vi "translate_to_from_byte_array.vi"(0 "actions":T1, 5 "byte_array (in)":u8[](array[numeric]), 7 "string (in)":string) -> (6 "byte_array (out)":u8[](array[numeric]), 8 "string (out)":string)   [LabVIEW 2013, in "common.lvlib"]
doc: "Converts a String to Byte Array and Byte Array to String for ease of communication with Performax hardware.\n\nProduced By:\n\n<B>Kod Integrations, LLC</B>\n4835 Marianne Drive\nMount Airy, MD 21771\nhttp://www.kodintegrations.com\nemail: info@kodintegrations.com\nphone: (240) 687-1288"
uses:
  common.lvlib
  translate_to_from_byte_array_actions.ctl
panel:
  in  "pre_init_bytearray (64 elements of 0)":u8[](array[numeric])=[0, 0, 0, 0, 0, 0, 0, 0, 0, 0, 0, 0, 0, 0, 0, 0, 0, 0, 0, 0, 0, 0, 0, 0, 0, 0, 0, 0, 0, 0, 0, 0, 0, 0, 0, 0, 0, 0, 0, 0, 0, 0, 0, 0, 0, 0, 0, 0, 0, 0, 0, 0, 0, 0, 0, 0, 0, 0, 0, 0, 0, 0, 0, 0]
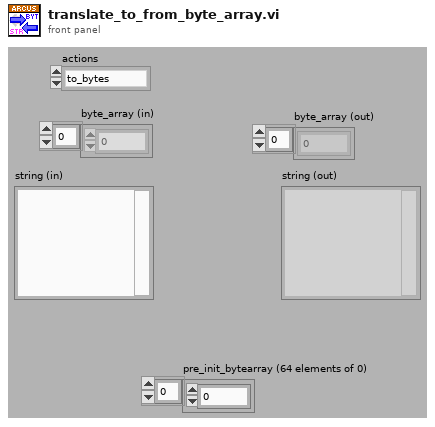
[diagram p1: front panel]
types:
  T1 = typedef "common.lvlib/translate_to_from_byte_array_actions.ctl" = enum16{"to_bytes", "to_string"}
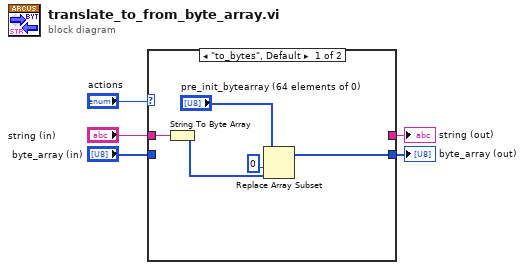
[diagram p0: block diagram]
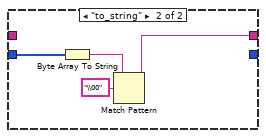
[diagram p2: hidden frame]
diagram:
  n1 = case shown="\"to_bytes\", Default" "actions" {
    tunnel: "string (in)" -> [w10 _]
    tunnel: "byte_array (in)" -> [_ w12]
    tunnel: [_ w11] -> w2
    tunnel: [w6 _] -> w1
    frame "to_bytes", Default {
      n2 = String To Byte Array(string=w10) -> (unsigned byte array=w7:u8[])
      n3 = Replace Array Subset(array="pre_init_bytearray (64 elements of 0)", new element=w7, index=0) -> (w6:u8[])
    }
    frame "to_string" {
      n4 = Byte Array To String(unsigned byte array=w12) -> (string=w14:string)
      n5 = Match Pattern(string=w14, regular expression="\\00") -> (before substring=w11:string)  [unwired: 1 in, 3 out]
    }
  }
  "byte_array (out)" <- w1
  "string (out)" <- w2
